vi "DecodeData.vi"(11 "Data In":u16[](array[numeric])) -> (0 "Current":i16[](array[numeric]), 1 "Toroidal":i16[](array[numeric]), 2 "Poloidal":i16[](array[numeric]), 3 "QRatio":i32[](array[numeric]), 4 "Flags":i16[](array[numeric]))   [LabVIEW 2009]
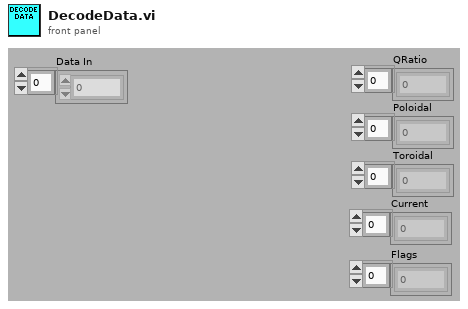
[diagram p1: front panel]
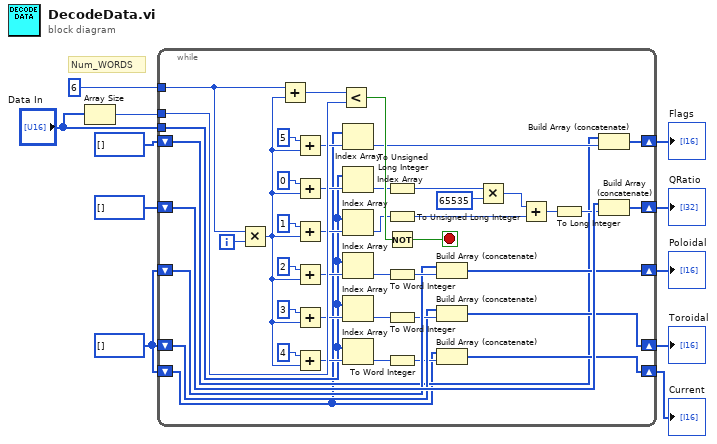
[diagram p0: block diagram]
diagram:
  w4 = i16[] [] ("Data Out")
  # "Num_WORDS"
  n1 = Array Size(array="Data In") -> (size(s)=w10:i32)
  n2 = while {
    tunnel: 6 -> [w52]
    tunnel: w10 -> [w53]
    shift-right: [w47] -> w9
    shift-left: i32[] [] ("Data Out") -> [w48]
    tunnel: "Data In" -> [w16]
    shift-right: [w31] -> w7
    shift-left: w4 -> [w32]
    shift-right: [w26] -> w5
    shift-left: w4 -> [w25]
    shift-right: [w17] -> w3
    shift-left: w4 -> [w13]
    shift-right: [w15] -> w1
    shift-left: u16[] [] ("Data Out") -> [w14]
    i -> [w56]
    stop <- w54 stop-if-true
    n3 = Multiply(x=w52, y=w56) -> (x*y=w12:i32)
    n4 = Add(x=w52, y=w12) -> (x+y=w51:i32)
    n5 = Add(x=5, y=w12) -> (x+y=w20:i32)
    n6 = Add(x=0, y=w12) -> (x+y=w50:i32)
    n7 = Add(x=1, y=w12) -> (x+y=w46:i32)
    n8 = Add(x=2, y=w12) -> (x+y=w36:i32)
    n9 = Add(x=3, y=w12) -> (x+y=w30:i32)
    n10 = Add(x=4, y=w12) -> (x+y=w24:i32)
    n11 = Less?(x=w51, y=w53) -> (x < y?=w55:bool)
    n12 = Index Array(array=w13, index=w20) -> (element=w18:i16)
    n13 = Index Array(array=w16, index=w50) -> (element=w43:u16)
    n14 = Index Array(array=w16, index=w46) -> (element=w41:u16)
    n15 = Index Array(array=w16, index=w36) -> (element=w34:u16)
    n16 = Index Array(array=w16, index=w30) -> (element=w28:u16)
    n17 = Index Array(array=w16, index=w24) -> (element=w22:u16)
    n18 = To Unsigned Long Integer(number=w43) -> (unsigned 32bit integer=w42:u32)
    n19 = To Unsigned Long Integer(number=w41) -> (unsigned 32bit integer=w40:u32)
    n20 = Not(x=w55) -> (.not. x?=w54:bool)
    n21 = To Word Integer(number=w34) -> (16bit integer=w33:i16)
    n22 = To Word Integer(number=w28) -> (16bit integer=w27:i16)
    n23 = To Word Integer(number=w22) -> (16bit integer=w21:i16)
    n24 = Build Array (concatenate)(w32, w33) -> (w31:i16[])
    n25 = Build Array (concatenate)(w25, w27) -> (w26:i16[])
    n26 = Build Array (concatenate)(w13, w21) -> (w17:i16[])
    n27 = Multiply(x=w42, y=u32 65535) -> (x*y=w44:u32)
    n28 = Add(x=w44, y=w40) -> (x+y=w39:u32)
    n29 = To Long Integer(number=w39) -> (32bit integer=w38:i32)
    n30 = Build Array (concatenate)(w14, w18) -> (w15:u16[])
    n31 = Build Array (concatenate)(w48, w38) -> (w47:i32[])
  }
  "QRatio" <- w9
  "Poloidal" <- w7
  "Toroidal" <- w5
  "Current" <- w3
  "Flags" <- w1
